vi "xps_panel_DO_set_stage_speed.vi"(8 "error in (no error)":errorcluster, 9 "stage_speed":dbl, 11 "newport_xps_panel in":refnum<class "newport_xps_panel.lvclass">) -> (0 "error out":errorcluster, 3 "newport_xps_panel out":refnum<class "newport_xps_panel.lvclass">)   [LabVIEW 2015, in "newport_xps_panel.lvclass"]
uses:
  newport_xps_panel.lvclass
  newport_xps/newport_xps.lvclass
  UI/panel_class/panel.lvclass
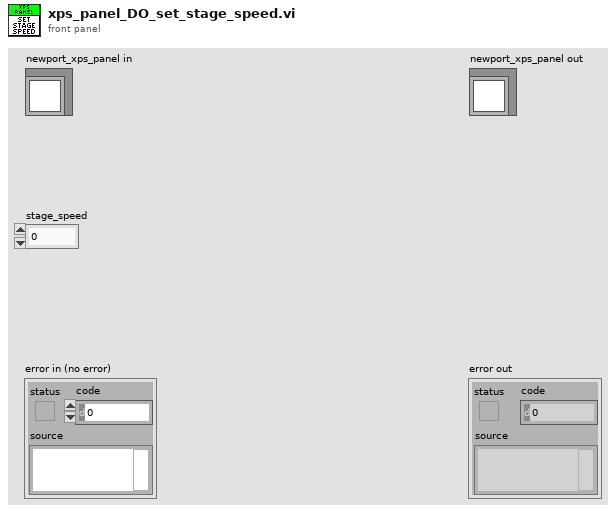
[diagram p1: front panel]
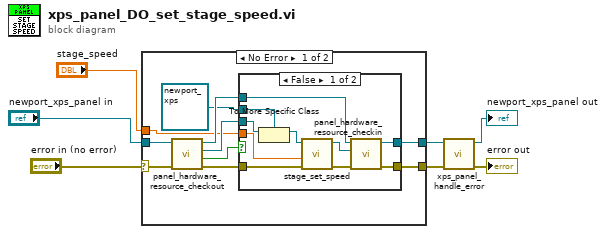
[diagram p0: block diagram]
diagram:
  n1 = case shown="No Error" "error in (no error)" {
    selector: "error in (no error)" -> [w16 w31]
    tunnel: [w12 w31] -> w4
    tunnel: [w11 w30] -> w3
    tunnel: "newport_xps_panel in" -> [w17 w30]
    tunnel: "stage_speed" -> [w8 _]
    frame No Error {
      n2 = call "panel_hardware_resource_checkout.vi"("error in (no error)"=w16, "panel in"=w17) -> ("error out"=w10:errorcluster, "timed out?"=w9:bool, "hardware.lvclass"=w13:refnum<class "hardware.lvclass">, "panel out"=w15:refnum<class "newport_xps_panel.lvclass">)  [unwired: 6 in]
      n3 = case shown="False" w9 {
        tunnel: w15 -> [w25 w29]
        tunnel: refnum<class "newport_xps.lvclass"> refnum ("newport_xps.lvclass") -> [w27 _]
        tunnel: w13 -> [w26 _]
        tunnel: [w24 w28] -> w12
        tunnel: [w23 w29] -> w11
        tunnel: w10 -> [w18 w28]
        tunnel: w8 -> [w19 _]
        frame False {
          n4 = To More Specific Class(target class=w27, reference=w26) -> (specific class reference=w22:refnum<class "newport_xps.lvclass">)  [unwired: 1 in, 1 out]
          n5 = call-dynamic "stage_set_speed.vi"("error in (no error)"=w18, "Speed"=w19, "newport_xps in"=w22) -> ("error out"=w20:errorcluster, "newport_xps out"=w21:refnum<class "newport_xps.lvclass">)  [unwired: 7 in]
          n6 = call "panel_hardware_resource_checkin.vi"("error in (no error)"=w20, "hardware.lvclass"=w21, "panel in"=w25) -> ("error out"=w24:errorcluster, "panel out"=w23:refnum<class "newport_xps_panel.lvclass">)  [unwired: 7 in]
        }
        frame True {
        }
      }
    }
    frame Error {
    }
  }
  n7 = call "xps_panel_handle_error.vi"("error in (no error)"=w4, "newport_xps_panel in"=w3) -> ("error out"=→"error out":errorcluster, "newport_xps_panel out"=→"newport_xps_panel out":refnum<class "newport_xps_panel.lvclass">)  [unwired: 8 in]
